vi "write_attributes.vi"(8 "error in (no error)":errorcluster, 10 "attributes":T1, 11 "ExtraTreeRegressor in":refnum<class "ExtraTreeRegressor.lvclass">) -> (0 "error out":errorcluster, 3 "ExtraTreeRegressor out":refnum<class "ExtraTreeRegressor.lvclass">)   [LabVIEW 2020, in "ExtraTreeRegressor.lvclass"]
uses:
  ExtraTreeRegressor.lvclass
  Controls/extra_tree_regressor_attributes.ctl
  ExtraTreeRegressor.lvclass/ExtraTreeRegressor.ctl
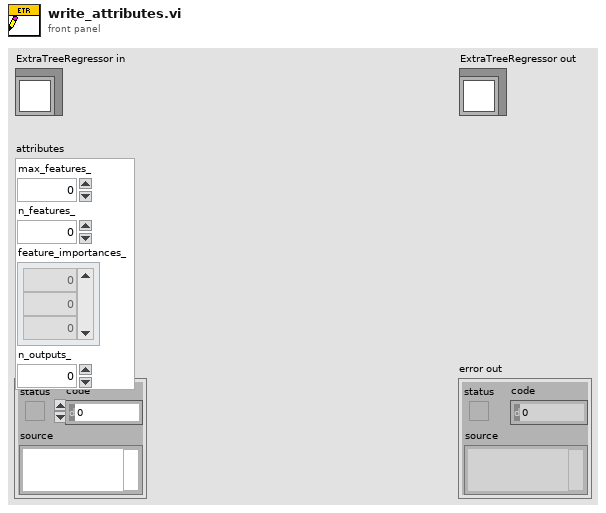
[diagram p1: front panel]
types:
  T1 = typedef "extra_tree_regressor_attributes.ctl" = cluster{"max_features_":dbl, "n_features_":dbl, "feature_importances_":dbl[], "n_outputs_":dbl}
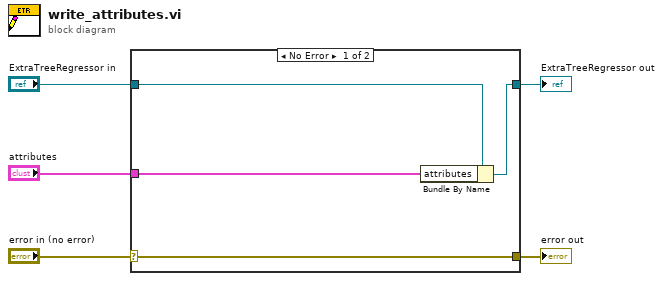
[diagram p0: block diagram]
diagram:
  n1 = case shown="No Error" "error in (no error)" {
    selector: "error in (no error)" -> [w9 w10]
    tunnel: [w9 w10] -> w4
    tunnel: [w7 w11] -> w2
    tunnel: "ExtraTreeRegressor in" -> [w8 w11]
    tunnel: "attributes" -> [w6 _]
    frame No Error {
      n2 = Bundle By Name(cluster=w8, "attributes"=w6) -> (w7:refnum<class "ExtraTreeRegressor.lvclass">)
    }
    frame Error {
    }
  }
  "error out" <- w4
  "ExtraTreeRegressor out" <- w2
